vi "FestoCPX.DI.Data.Get.vi"   [LabVIEW 2013]
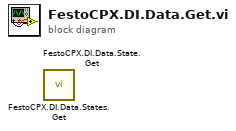
[diagram p0: block diagram]
diagram:
  n1 = call "FestoCPX.DI.Data.States.Get.vi"() -> ()  [unwired: 10 in, 2 out]
  n2 = call "FestoCPX.DI.Data.State.Get.vi"() -> ()  [unwired: 10 in, 2 out]
